vi "Stop.vi"(8 "error in (no error)":errorcluster, 11 "JQMHCore in":refnum<class "Module.lvclass">) -> (0 "error out":errorcluster)   [LabVIEW 2024, in "Module.lvclass"]
uses:
  Module.lvclass
  Module.lvclass/Module.ctl
  StopEventArgs.ctl
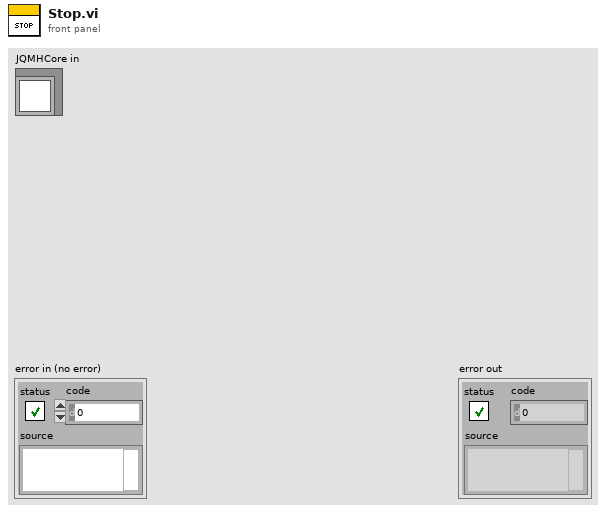
[diagram p1: front panel]
types:
  T1 = typedef "Module.lvclass/StopEventArgs.ctl" = bool
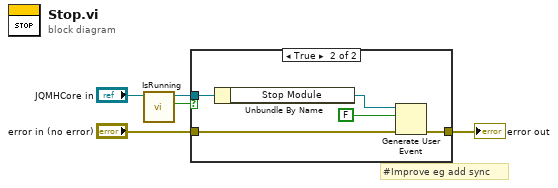
[diagram p0: block diagram]
diagram:
  # "#Improve eg add sync"
  n1 = call "IsRunning.vi"("JQMHModule in"="JQMHCore in") -> ("Is Running?"=w3:bool, "JQMHModule out"=w1:refnum<class "Module.lvclass">)  [unwired: 9 in]
  n2 = case shown="True" w3 {
    tunnel: "error in (no error)" -> [w6 w10]
    tunnel: [w6 w9] -> w4
    tunnel: w1 -> [_ w7]
    frame False {
    }
    frame True {
      n3 = Unbundle By Name(w7) -> ("Stop Module"=w11:refnum<user-event>)
      n4 = Generate User Event(user event=w11, event data cluster=T1 FALSE ("event data"), error in=w10) -> (error out=w9:errorcluster)  [unwired: 1 in, 1 out]
    }
  }
  "error out" <- w4
